vi "Measure Frame Rate.vi"() -> (2 "Frame Rate [FPS]":dbl format="%.0p", 3 "Delta Time [s]":dbl format="%.0p")   [LabVIEW 2022 SP3, in "Utility.lvlib"]
uses:
  Utility.lvlib
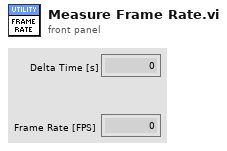
[diagram p1: front panel]
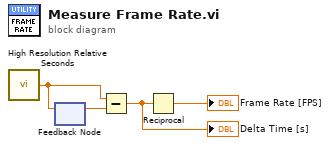
[diagram p0: block diagram]
diagram:
  n1 = call <vilib>:"High Resolution Relative Seconds.vi"() -> ("relative seconds"=w4:dbl)
  n2 = feedback #1() -> (w3:dbl)  [unwired: 1 in]
  n3 = feedback-in #1(w4) -> ()
  n4 = Subtract(x=w4, y=w3) -> (x-y=w2:dbl)
  "Delta Time [s]" <- w2
  n5 = Reciprocal(x=w2) -> (1/x=→"Frame Rate [FPS]":dbl)
